vi "VI Owning Palette.vi"(0 "Destination":path=path "") -> (1 "Name":string, 2 "URL":string)   [LabVIEW 2018, in "Scripts.lvlib"]
uses:
  Scripts.lvlib
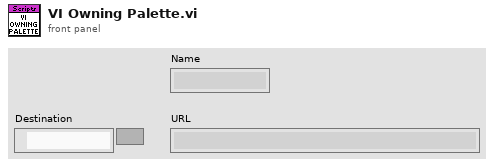
[diagram p1: front panel]
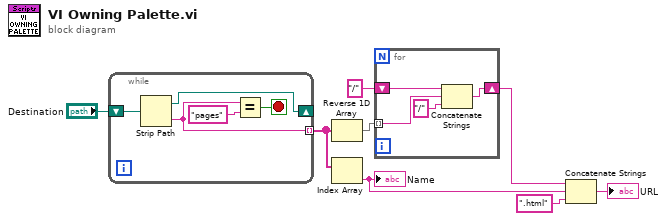
[diagram p0: block diagram]
diagram:
  n1 = while {
    shift-right: [w10] -> _
    shift-left: "Destination" -> [w13]
    tunnel: [w9] -> w5 mode=indexing
    stop <- w11 stop-if-true
    n2 = Strip Path(path=w13) -> (stripped path=w10:path, name=w9:string)
    n3 = Equal?(x=w9, y="pages") -> (x = y?=w11:bool)
  }
  n4 = Reverse 1D Array(array=w5) -> (reversed array=w2:string[])
  n5 = Index Array(array=w5) -> (element=w8:string)  [unwired: 1 in]
  "Name" <- w8
  n6 = for {
    tunnel: w2 -> [w16] mode=indexing
    shift-right: [w14] -> w4
    shift-left: "/" -> [w17]
    n7 = Concatenate Strings(w17, w16, "/") -> (w14:string)
  }
  n8 = Concatenate Strings(w4, w8, ".html" ("string")) -> (→"URL":string)
